vi "PH_Beckhoff-16BB.set i Attr and start DIM Services.vi"(0 "i ref in":refnum<vi>, 2 "Values":T6, 3 "Racktype":string, 5 "error in":errorcluster) -> (14 "i ref out":refnum<vi>, 17 "i Attr":T1={"PA Chiller"={"PSDB"={"Status Service ID"=-1, "Instance ID"=-1, "Data Status"=0, "Ref Status"=refnum, "Error Code"=0}, "Status"={"GUI Ref"=refnum, "Status Service ID"=-1, "Status"=0}, "DIs"={"Flow Control"={"GUI Ref"=refnum, "# in Data"=-1}, "High-Temp"={"GUI Ref"=refnum, "# in Data"=-1}, "Conductivity"={"GUI Ref"=refnum, "# in Data"=-1}, "Niveau"={"GUI Ref"=refnum, "# in Data"=-1}}, "PSDB Thread"={"Ref"=refnum, "Q-Ref"=refnum}}, "PSDB"={"Shot #"=-1, "Subsystem"=0}, "Racktype"="", "PSDB Credentials"={"PW"="N/A", "ID"="N/A", "DS"="N/A"}} {"PSDB"."Subsystem" items=["Miscellaneous", "fs-Frontend", "ns-Frontend", "PreAmp", "MainAmp", "MAS", "COS", "Beamline", "Experiment Laserbay", "Experiment Laserlabor", "Experiment Z6", "Timing", "Pulsed Power"]; "PA Chiller"."Status"."Status" items=["no info", "off/false/out", "on/true/in", "Failure", "Alarm", "Status 1", "Status 2", "Status 3"]; "PA Chiller"."PSDB"."Data Status" items=["no info", "no Data collection", "no problem", "Error getting the ID", "Error writing Data", "Error getting the subsystem", "Error getting the Shot ID", "Error getting the Shot Types", "Error getting the Experiments", "Error verifying wanted Shottype", "Error verifying wanted Experiment"]}, 19 "error out":errorcluster)   [LabVIEW 2014, in "PH_Beckhoff-16BB.lvlib"]
doc: "This VI gets the # of relevant data in the related data array(s) and stores them at own attributes."
uses:
  PH_Beckhoff-16BB.lvlib
  PH_Beckhoff/PH_Beckhoff.Values.ctl
  PH_Beckhoff/PH_Beckhoff.Sonderklemmen Inputs.ctl
  PH_Beckhoff/PH_Beckhoff.Analog Inputs.ctl
  PH_Beckhoff/PH_Beckhoff.Scaling Type.ctl
  PH_Beckhoff/PH_Beckhoff.Analog Outputs.ctl
  PH_Beckhoff/PH_Beckhoff.Digital Inputs.ctl
  PH_Beckhoff/PH_Beckhoff.Digital Outputs.ctl
  PH_Beckhoff-16BB.i attribute.ctl
  PH_Basics/PH_PSDBWriter/PH_PSDBWriter.Data Status.ctl
  PH_Basics/PH_StatusHandler/PH_StatusHandler.Status.ctl
  PH_Basics/PH_PSDBWriter/PH_PSDBWriter.PHELIX-Subsystems.ctl
  PH_Basics/PH_Common/Connection/PH_Connection.PSDB Credentials.ctl
  PH_Beckhoff-16BB.PA Chiller Tags.ctl
  PH_Basics/PH_PSDBWriter/PH_PSDBWriter.lvlib
  PH_Basics/PH_StatusHandler/PH_StatusHandler.lvlib
  CSlibraries-extern/DimLVEvent/LVDimInterface/LVDimInterface.lvlib
  CS_Core/CSSystem/CSSystemLib/CSSystemLib.lvlib
  PH_Basics/PH_Common/PH_Common.lvlib
  PH_Beckhoff/PH_Beckhoff.lvlib
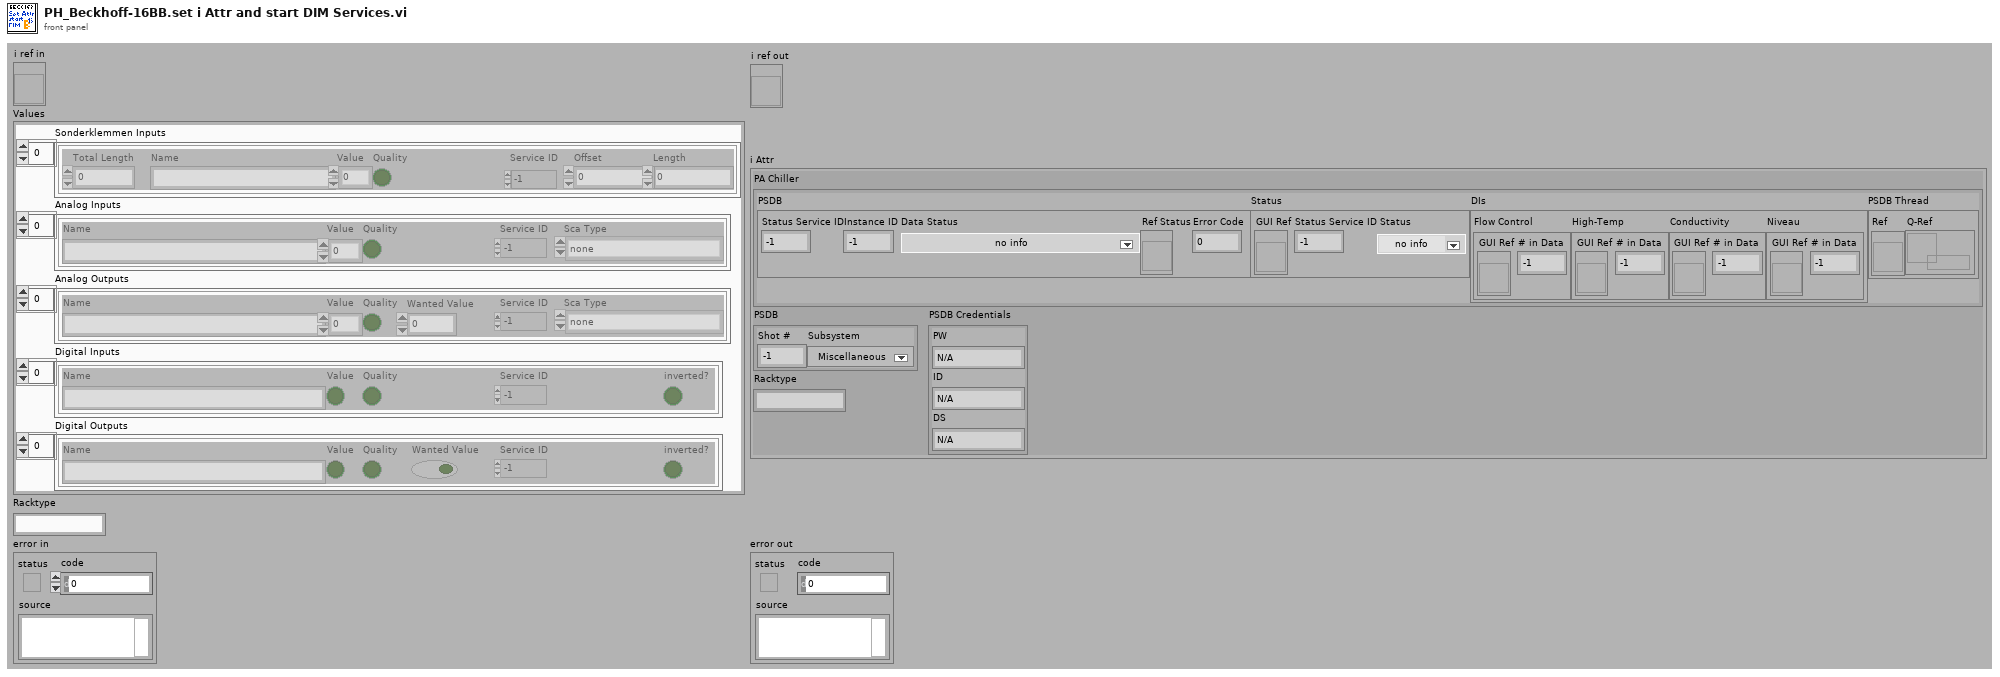
[diagram p1: front panel]
types:
  T1 = typedef "PH_Beckhoff-16BB.lvlib/PH_Beckhoff-16BB.i attribute.ctl" = cluster{"PA Chiller":cluster{"PSDB":cluster{"Status Service ID":i32, "Instance ID":i32, "Data Status":T2, "Ref Status":refnum<vi>, "Error Code":i32}, "Status":cluster{"GUI Ref":refnum<vi>, "Status Service ID":i32, "Status":T3}, "DIs":cluster{"Flow Control":cluster{"GUI Ref":refnum<vi>, "# in Data":i32}, "High-Temp":cluster{"GUI Ref":refnum<vi>, "# in Data":i32}, "Conductivity":cluster{"GUI Ref":refnum<vi>, "# in Data":i32}, "Niveau":cluster{"GUI Ref":refnum<vi>, "# in Data":i32}}, "PSDB Thread":cluster{"Ref":refnum<vi>, "Q-Ref":refnum<queue>}}, "PSDB":cluster{"Shot #":i32, "Subsystem":T4}, "Racktype":string, "PSDB Credentials":T5}
  T2 = typedef "PH_PSDBWriter.lvlib/PH_PSDBWriter.Data Status.ctl" = i16
  T3 = typedef "PH_StatusHandler.lvlib/PH_StatusHandler.Status.ctl" = i16
  T4 = typedef "PH_PSDBWriter.lvlib/PH_PSDBWriter.PHELIX-Subsystems.ctl" = i32
  T5 = typedef "PH_Common.lvlib/PH_Connection.PSDB Credentials.ctl" = cluster{"PW":string, "ID":string, "DS":string}
  T6 = typedef "PH_Beckhoff.lvlib/PH_Beckhoff.Values.ctl" = cluster{"Sonderklemmen Inputs":T7, "Analog Inputs":T8, "Analog Outputs":T10, "Digital Inputs":T11, "Digital Outputs":T12}
  T7 = typedef "PH_Beckhoff.lvlib/PH_Beckhoff.Sonderklemmen Inputs.ctl" = cluster{"Total Length":u32, "Name":string, "Value":u64, "Quality":bool, "Service ID":i32, "Offset":u32, "Length":u32}[]
  T8 = typedef "PH_Beckhoff.lvlib/PH_Beckhoff.Analog Inputs.ctl" = cluster{"Name":string, "Value":u32, "Quality":bool, "Service ID":i32, "Sca Type":T9}[]
  T9 = typedef "PH_Beckhoff.lvlib/PH_Beckhoff.Scaling Type.ctl" = enum16{"none", "0 ... 15 Bit -> 0 ... 5", "0 ... 15 Bit -> 0 ... 10", "0 ... 15 Bit -> 0 ... 25", "0 ... 15 Bit -> 4 ... 20", "0 ... 15 Bit -> 0 ... 1", "0 ... 15 Bit -> 0 ... 20000", "0 ... 15 Bit -> 0 ... 24000"}
  T10 = typedef "PH_Beckhoff.lvlib/PH_Beckhoff.Analog Outputs.ctl" = cluster{"Name":string, "Value":u32, "Quality":bool, "Wanted Value":u32, "Service ID":i32, "Sca Type":T9}[]
  T11 = typedef "PH_Beckhoff.lvlib/PH_Beckhoff.Digital Inputs.ctl" = cluster{"Name":string, "Value":bool, "Quality":bool, "Service ID":i32, "inverted?":bool}[]
  T12 = typedef "PH_Beckhoff.lvlib/PH_Beckhoff.Digital Outputs.ctl" = cluster{"Name":string, "Value":bool, "Quality":bool, "Wanted Value":bool, "Service ID":i32, "inverted?":bool}[]
  T13 = typedef "PH_Beckhoff-16BB.lvlib/PH_Beckhoff-16BB.PA Chiller Tags.ctl" = enum16{"Flow-control", "High-temp", "Conductivity", "Niveau", "Status"}
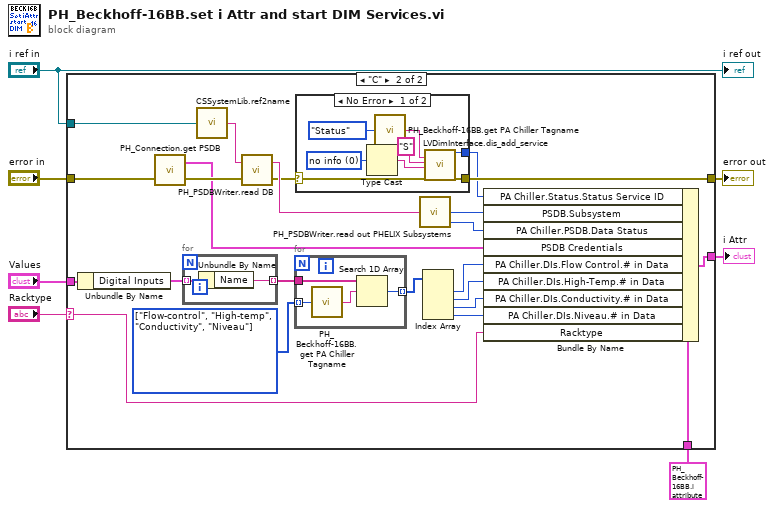
[diagram p0: block diagram]
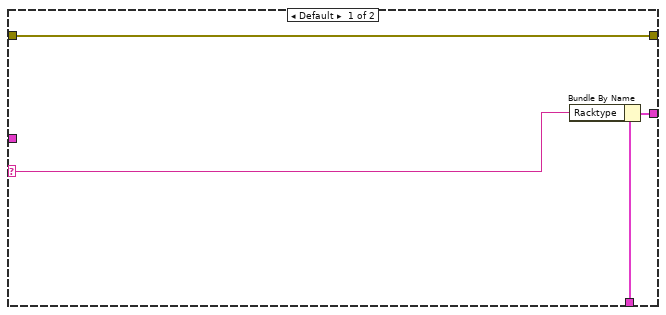
[diagram p2: hidden frame]
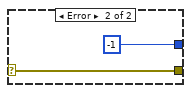
[diagram p3: hidden frame]
diagram:
  n1 = case shown="\"C\"" "Racktype" {
    selector: "Racktype" -> [w8 w16]
    tunnel: "Values" -> [_ w31]
    tunnel: T1 {"PA Chiller"={"PSDB"={"Status Service ID"=-1, "Instance ID"=-1, "Data Status"=0, "Ref Status"=refnum, "Error Code"=0}, "Status"={"GUI Ref"=refnum, "Status Service ID"=-1, "Status"=0}, "DIs"={"Flow Control"={"GUI Ref"=refnum, "# in Data"=-1}, "High-Temp"={"GUI Ref"=refnum, "# in Data"=-1}, "Conductivity"={"GUI Ref"=refnum, "# in Data"=-1}, "Niveau"={"GUI Ref"=refnum, "# in Data"=-1}}, "PSDB Thread"={"Ref"=refnum, "Q-Ref"=refnum}}, "PSDB"={"Shot #"=-1, "Subsystem"=0}, "Racktype"="", "PSDB Credentials"={"PW"="N/A", "ID"="N/A", "DS"="N/A"}} ("i attribute") -> [w10 w25]
    tunnel: "error in" -> [w11 w24]
    tunnel: [w11 w22] -> w4
    tunnel: "i ref in" -> [_ w19]
    tunnel: [w9 w17] -> w2
    frame Default {
      n2 = Bundle By Name(cluster=w10, "Racktype"=w8) -> (w9:T1)
    }
    frame "C" {
      w32 = T13[] [enum."Flow-control", enum."High-temp", enum."Conductivity", enum."Niveau"] items=["Flow-control", "High-temp", "Conductivity", "Niveau", "Status"]
      n3 = Unbundle By Name(w31) -> ("Digital Inputs"=w33:T11)
      n4 = call "PH_Connection.get PSDB.vi"("error in (no error)"=w24) -> ("error out"=w13:errorcluster, "PSDB Credentials"=w12:T5)  [unwired: 1 in]
      n5 = for {
        tunnel: w33 -> [w46] mode=indexing
        tunnel: [w45] -> w34 mode=indexing
        n6 = Unbundle By Name(w46) -> ("Name"=w45:string)
      }
      n7 = call "CSSystemLib.ref2name.vi"("obj refnum"=w19) -> ("name"=w18:string)
      n8 = call "PH_PSDBWriter.read DB.vi"("error in"=w13, "Instance Name"=w18) -> ("error out"=w15:errorcluster, "PSDB Subsystem"=w20:string)
      n9 = for {
        tunnel: w32 -> [w50] mode=indexing
        tunnel: w34 -> [w49]
        tunnel: [w47] -> w30 mode=indexing
        n10 = call "PH_Beckhoff-16BB.get PA Chiller Tagname.vi"("PA Chiller Tag"=w50) -> ("PA Chiller Tagname"=w48:string)
        n11 = Search 1D Array(1D array=w49, element=w48) -> (index of element=w47:i32)  [unwired: 1 in]
      }
      n12 = case shown="No Error" w15 {
        selector: w15 -> [w40 w44]
        tunnel: [w42 -1 ("my_serviceID")] -> w21
        tunnel: [w41 w44] -> w22
        frame No Error {
          w35 = T3 0 items=["no info", "off/false/out", "on/true/in", "Failure", "Alarm", "Status 1", "Status 2", "Status 3"] ("Status")
          n13 = Type Cast(x=w35) -> (*(type *) &x=w39:string)  [unwired: 1 in]
          n14 = call "PH_Beckhoff-16BB.get PA Chiller Tagname.vi"("PA Chiller Tag"=PH_Beckhoff-16BB.PA_Chiller_Tags."Status") -> ("PA Chiller Tagname"=w37:string)
          n15 = call "LVDimInterface.dis_add_service.vi"("serviceName"=w37, "typeDescriptor"="S", "data"=w39, "error in (no error)"=w40) -> ("my_serviceID"=w42:i32, "error out"=w41:errorcluster)  [unwired: 14 in]
        }
        frame Error {
        }
      }
      n16 = call "PH_PSDBWriter.read out PHELIX Subsystems.vi"("Config DB Subsystem"=w20) -> ("Metadata.Data Status"=w14:T2, "Metadata.Subsystem"=w23:T4)  [unwired: 2 in, 1 out]
      n17 = Index Array(array=w30) -> (element #1=w29:i32, element #2=w28:i32, element #3=w27:i32, element #4=w26:i32)  [unwired: 4 in]
      n18 = Bundle By Name(cluster=w25, "PA Chiller.Status.Status Service ID"=w21, "PSDB.Subsystem"=w23, "PA Chiller.PSDB.Data Status"=w14, "PSDB Credentials"=w12, "PA Chiller.DIs.Flow Control.# in Data"=w29, "PA Chiller.DIs.High-Temp.# in Data"=w28, "PA Chiller.DIs.Conductivity.# in Data"=w27, "PA Chiller.DIs.Niveau.# in Data"=w26, "Racktype"=w16) -> (w17:T1)
    }
  }
  "error out" <- w4
  "i Attr" <- w2
  "i ref out" <- "i ref in"
